vi "MC_VERSION.vi"() -> (0 "MC Version":string)   [LabVIEW 2014]
doc: "Contains the version of the software to display on GUIs.\n\n\nAuthor: Mike Schultz"
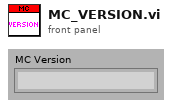
[diagram p1: front panel]
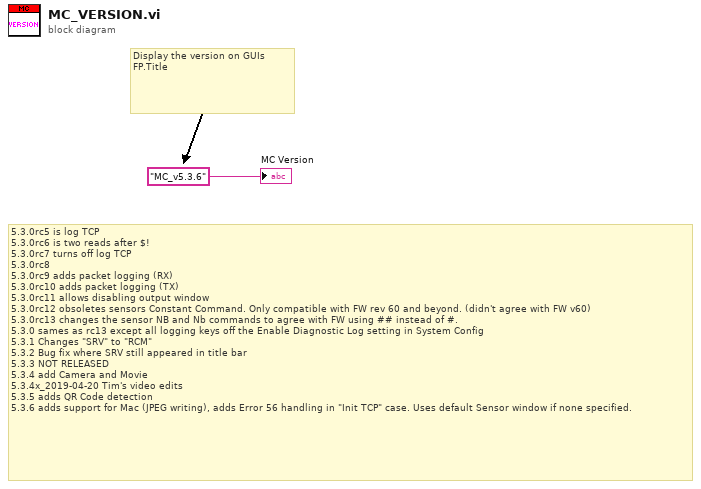
[diagram p0: block diagram]
diagram:
  # "5.3.0rc5 is log TCP\n5.3.0rc6 is two reads after $!\n5.3.0rc7 turns off log TCP\n5.3.0rc8\n5.3.0rc9 adds packet logging (RX)\n5.3.0rc10 adds packet logging (TX)\n5.3.0rc11 allows disabling output window\n5.3.0rc12 obsoletes sensors Constant Command. Only compatible with FW rev 60 and beyond. (didn't agree with FW v60)\n5.3.0rc13 changes the sensor NB and Nb commands to agree with FW using ## instead of #.\n5.3.0 sames as rc13 except all logging keys off the Enable Diagnostic Log setting in System Config\n5.3.1 Changes \"SRV\" to \"RCM\"\n5.3.2 Bug fix where SRV still appeared in title bar\n5.3.3 NOT RELEASED\n5.3.4 add Camera and Movie\n5.3.4x_2019-04-20 Tim's video edits\n5.3.5 adds QR Code detection\n5.3.6 adds support for Mac (JPEG writing), adds Error 56 handling in \"Init TCP\" case. Uses default Sensor window if none specified."
  # "Display the version on GUIs\nFP.Title"
  "MC Version" <- "MC_v5.3.6" ("Front Panel Window:Title")
